vi "Do.vi"(8 "error in (no error)":errorcluster, 10 "Msg Queue":refnum<queue>, 11 "State Cmd in":refnum<class "Stop Msg.lvclass">=refnum) -> (0 "error out":errorcluster, 3 "State Cmd out":refnum<class "Stop Msg.lvclass">)   [LabVIEW 2020, in "OOP SM.lvlib" / "Stop Msg.lvclass"]
uses:
  Stop Msg.lvclass
  Message/Message.lvclass
  <vilib>/Utility/error.llb/Error Cluster From Error Code.vi
  <vilib>/ErrorRing/Error Ring.xnode
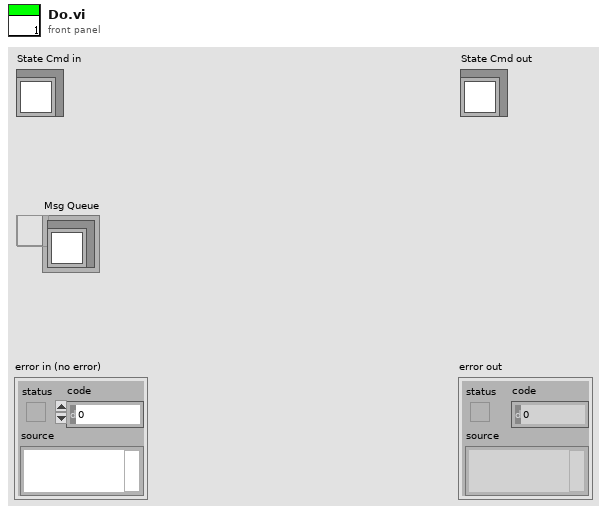
[diagram p1: front panel]
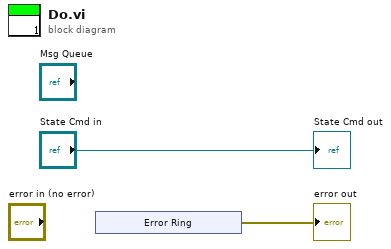
[diagram p0: block diagram]
diagram:
  n1 = xnode "Error Ring"() -> ("error out"=→"error out":errorcluster)
  "State Cmd out" <- "State Cmd in"
